vi "gaussmeter read polar.vi"(8 "error in (no error)":errorcluster, 11 "VISA resource name":refnum<visa-resource-name>="GPIB1::11::INSTR") -> (0 "error out":errorcluster, 2 "magnet polar":T1, 3 "VISA resource name 2":refnum<visa-resource-name>)   [LabVIEW 2013]
uses:
  magnet/magnet polar field.ctl
  app/app global state actions.ctl
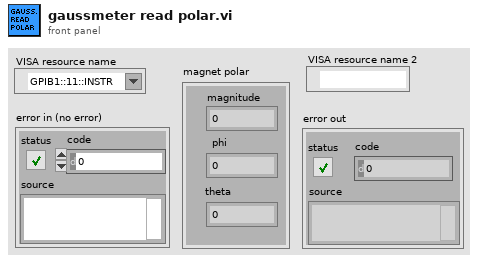
[diagram p1: front panel]
types:
  T1 = typedef "magnet polar field.ctl" = cluster{"magnitude":dbl, "phi":dbl, "theta":dbl}
  T2 = typedef "app global state actions.ctl" = enum16{"set field reached", "get cluster", "set cluster", "set current sweep", "set field value", "set 430 TCP reading", "set ramping", "set sweeping", "append log", "clear log", "set finished"}
  T3 = typedef "magnet cartesian field.ctl" = cluster{"X (T)":dbl, "Y (T)":dbl, "Z (T)":dbl, "Magnitude (T)":dbl}
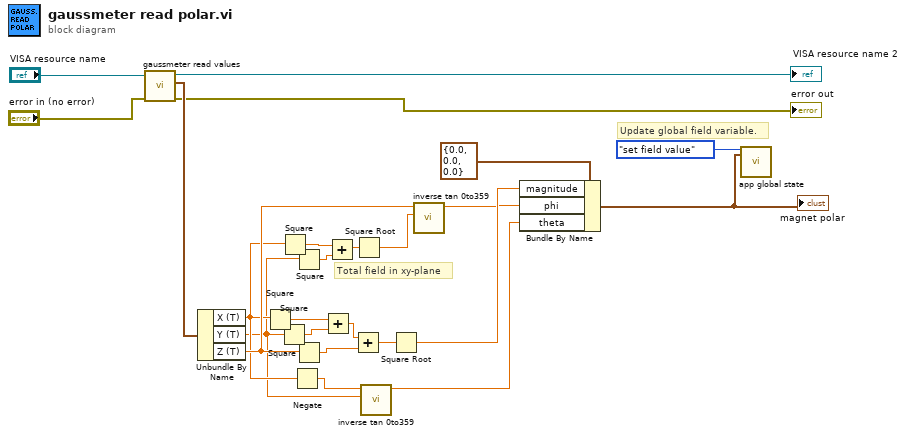
[diagram p0: block diagram]
diagram:
  # "Total field in xy-plane"
  # "Update global field variable."
  n1 = call "gaussmeter read values.vi"("error in (no error)"="error in (no error)", "VISA resource name"="VISA resource name") -> ("error out"=→"error out":errorcluster, "gaussmeter reading"=w22:T3, "VISA resource name"=→"VISA resource name 2":refnum<visa-resource-name>)  [unwired: 7 in]
  n2 = Unbundle By Name(w22) -> ("X (T)"=w2:dbl, "Y (T)"=w1:dbl, "Z (T)"=w10:dbl)
  n3 = Square(x=w2) -> (x^2=w18:dbl)
  n4 = Square(x=w1) -> (x^2=w17:dbl)
  n5 = Square(x=w2) -> (x^2=w6:dbl)
  n6 = Negate(x=w2) -> (-x=w8:dbl)
  n7 = Square(x=w1) -> (x^2=w5:dbl)
  n8 = Square(x=w10) -> (x^2=w15:dbl)
  n9 = Add(x=w18, y=w17) -> (x+y=w16:dbl)
  n10 = Add(x=w6, y=w5) -> (x+y=w3:dbl)
  n11 = Add(x=w16, y=w15) -> (x+y=w14:dbl)
  n12 = Square Root(x=w3) -> (sqrt(x)=w4:dbl)
  n13 = call "inverse tan 0to359.vi"("y coil"=w1, "z coil"=w8) -> ("phi (deg)"=w9:dbl)  [unwired: 9 in]
  n14 = Square Root(x=w14) -> (sqrt(x)=w11:dbl)
  n15 = call "inverse tan 0to359.vi"("y coil"=w4, "z coil"=w10) -> ("phi (deg)"=w7:dbl)  [unwired: 9 in]
  n16 = Bundle By Name(cluster=T1 {"magnitude"=0.0, "phi"=0.0, "theta"=0.0} ("magnet polar"), "magnitude"=w11, "phi"=w7, "theta"=w9) -> (w12:T1)
  "magnet polar" <- w12
  n17 = call "app global state.vi"("action"=app_global_state_actions."set field value", "magnet polar"=w12) -> ()  [unwired: 17 in, 1 out]
